vi "132CAM2 side.vi"() -> ()   [LabVIEW 2015]
uses:
  <vilib>/Platform/TimedLoop/XDataNode/timing_clust.ctl
  <vilib>/Platform/TimedLoop/XDataNode/nitl_modes.ctl
  <vilib>/Platform/TimedLoop/XDataNode/wakeup.ctl
  <vilib>/platform/TimedLoop/XDataNode/XDataNode.xnode
  <vilib>/Platform/TimedLoop/XDataNode/XDNodeRunTimeDep.lvlib
  <vilib>/vision/NI_Vision_Development_Module.lvlib
panel:
  out "APX HPC SIDE 2":T1(plugin-control)
  out "Coordinates":i32[](array[numeric])
  out "Line Profile":cluster{"x0":sgl, "dx":sgl, "Pixels Line":sgl[]}(graph)
  out "Line Information":T2 {"Standard Deviation" format="%#.2f"; "Mean" format="%#.2f"}
  out "APX HPC SIDE":T1(plugin-control)
  out "APX HPC SIDE":T1(plugin-control)
  in  "stop":bool
  # "26u/pixel"
  # "0.5mm"
  # "12mm"
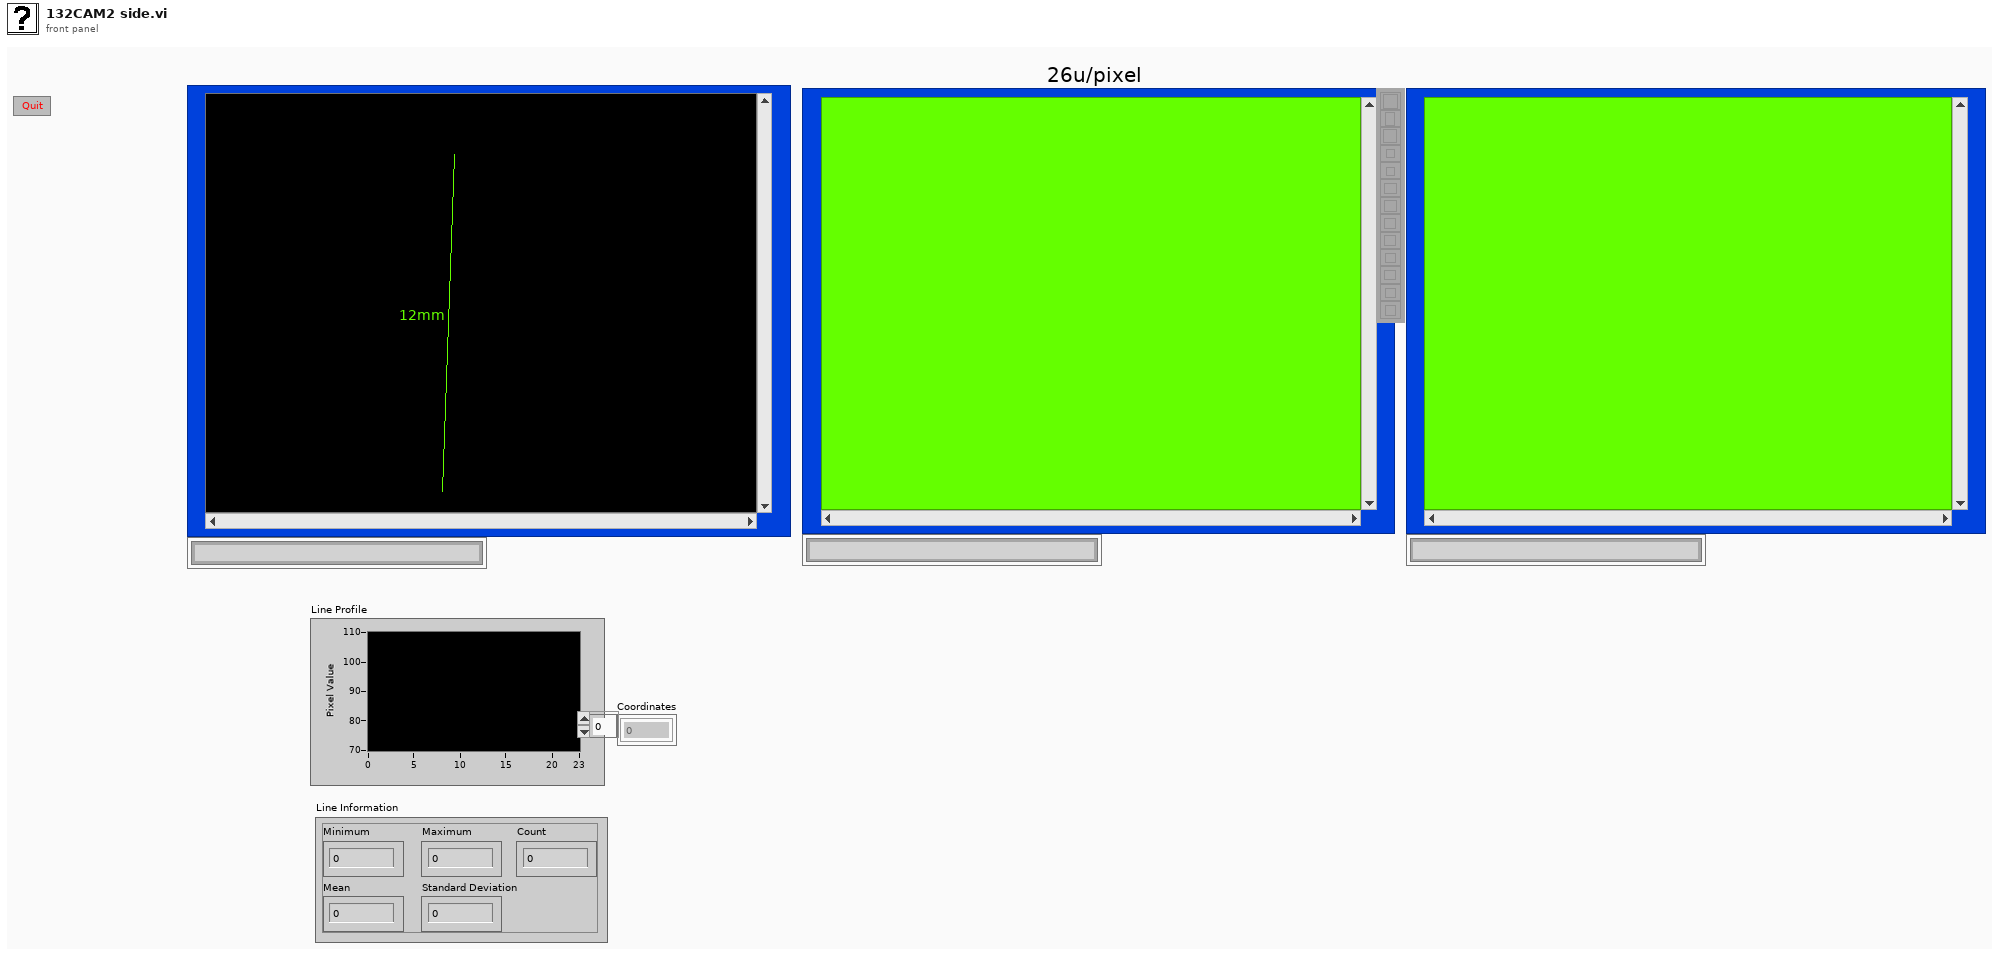
[diagram p1: front panel]
types:
  T1 = typedef "IMAQ Image.ctl" = refnum<image>
  T2 = cluster{"Minimum":sgl, "Maximum":sgl, "Mean":sgl, "Standard Deviation":sgl, "Count":i32}
  T3 = typedef "XDNodeRunTimeDep.lvlib/timing_clust.ctl" = cluster{"Expected End [f-1]":u64, "Actual End [f-1]":u64, "Finished Late? [f-1]":bool, "Expected End [i-1]":u64, "Actual End [i-1]":u64, "Finished Late? [i-1]":bool, "Expected Start [i]":u64, "Actual Start [i]":u64, "Expected Start [f]":u64, "Actual Start [f]":u64, "Source Name":string, "Structure Name":string, "Period":i64, "Deadline":i64, "Offset":i64, "Start":i64, "Priority":i32, "Timeout":i32, "Mode":T4, "Wakeup Reason":T5, "Error":errorcluster, "Source Type":string, "Secondary Source Type":string, "Global End Time":u64, "Global Start Time":u64, "Frame Duration":u64, "Iteration Duration":u64, "Assigned CPU":i32, "I/O Scan Engine Mode":u32}
  T4 = typedef "XDNodeRunTimeDep.lvlib/nitl_modes.ctl" = enum32{"No Change", "Process missed periods, maintain original phase", "Discard missed periods, maintain original phase", "Process missed periods, ignore original phase", "Discard missed periods, ignore original phase"}
  T5 = typedef "XDNodeRunTimeDep.lvlib/wakeup.ctl" = enum32{"Normal", "Aborted", "Asynchronous wakeup", "Timing source error", "Timed loop error", "Timeout"}
  T6 = cluster{"Min":sgl, "Max":sgl, "Mean":sgl, "Std Dev":sgl, "Count":i32}
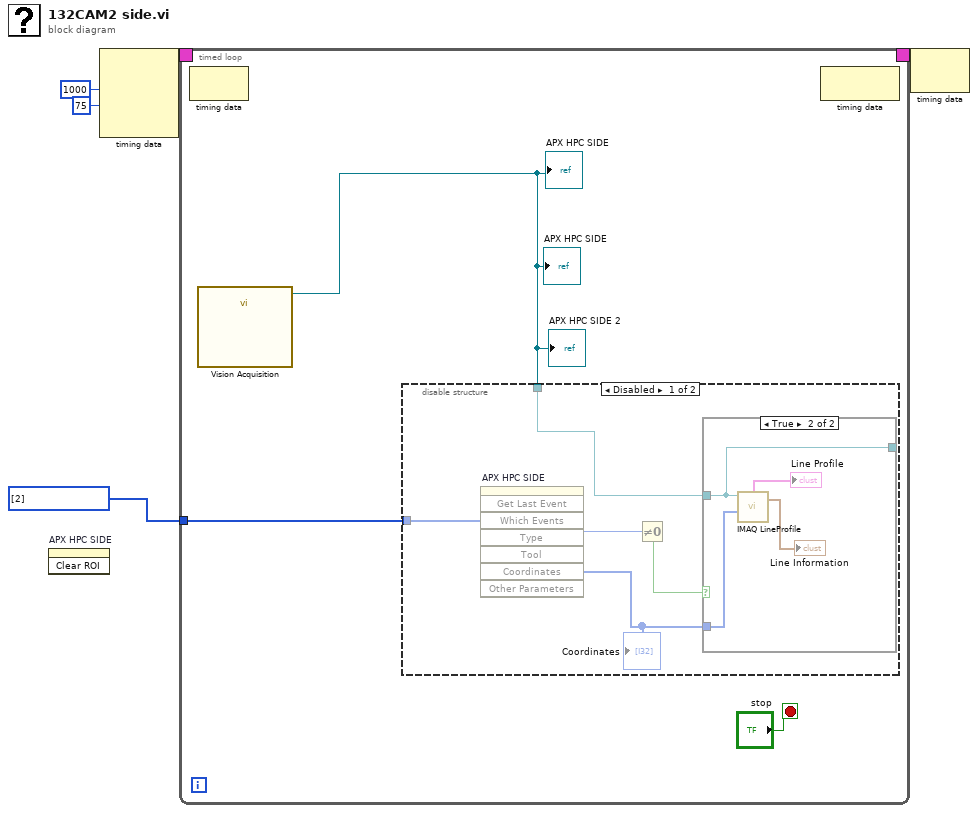
[diagram p0: block diagram]
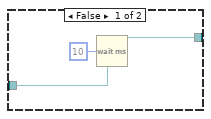
[diagram p2: hidden frame]
diagram:
  w1 = i32[] [2] items=["No  event", "Click event", "Draw event", "Move event", "Size event", "Scroll event", "Activate event", "Close event", "Double click event"] ("Events list (all)")
  n1 = invoke on="APX HPC SIDE" class="ImageControl" method="Clear ROI"() -> ()  [unwired: 3 in, 3 out]
  n2 = node-c288(i64 1000 ("Period"), 75 ("Priority")) -> (w5:T3)  [unwired: 2 in]
  n3 = timed-loop {
    timing: w5 -> [_]
    timing-out: [_] -> w4
    tunnel: w1 -> [w7]
    stop <- "stop" stop-if-true
    n4 = node-c288() -> ()  [unwired: 1 in, 1 out]
    n5 = call "Vision Acquisition"() -> ("Image Out"=w6:T1)  [unwired: 25 in, 2 out]
    "APX HPC SIDE" <- w6
    "APX HPC SIDE" <- w6
    "APX HPC SIDE 2" <- w6
    n6 = disable-structure shown="Disabled" {
      disable-tunnel: w7 -> [w10 _]
      disable-tunnel: w6 -> [w9 _]
      frame Disabled {
        n7 = invoke on="APX HPC SIDE" class="ImageControl" method="Get Last Event"("Which Events"=w10) -> ("Type"=w13:i32, "Coordinates"=w12:i32[])  [unwired: 7 in, 6 out]
        "Coordinates" <- w12
        n8 = Not Equal To 0?(x=w13) -> (x != 0?=w11:bool)
        n9 = case shown="True" w11 {
          tunnel: w9 -> [w14 w18]
          tunnel: [w14 w18] -> _
          tunnel: w12 -> [_ w19]
          frame False {
            n10 = Wait (ms)(milliseconds to wait=u32 10) -> ()  [unwired: 1 out]
          }
          frame True {
            n11 = call "IMAQ LineProfile"("Line Coordinates"=w19, "Image"=w18) -> ("Line Graph"=→"Line Profile":cluster{"x0":sgl, "dx":sgl, "Pixels Line":sgl[]}, "Line Information"=→"Line Information":T6)  [unwired: 3 in, 2 out]
          }
        }
      }
      frame Enabled {
      }
    }
    n12 = node-c288() -> ()  [unwired: 1 in, 1 out]
  }
  n13 = node-c288(w4) -> ()  [unwired: 1 out]
